vi "Us2.vi"() -> ()   [LabVIEW 2021]
panel:
  in  "\\hat b_min":dbl
  out "Us2":dbl
  out "error out":errorcluster
  in  "error in (no error)":errorcluster
  in  "z":dbl
  in  "eps":dbl
  in  "h":dbl
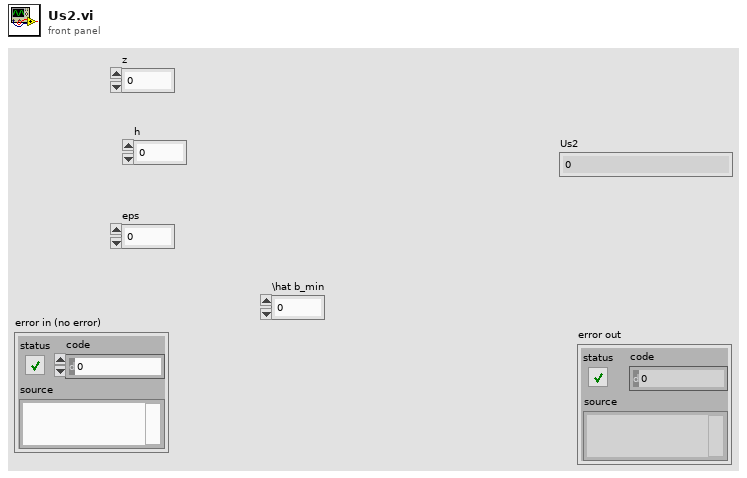
[diagram p1: front panel]
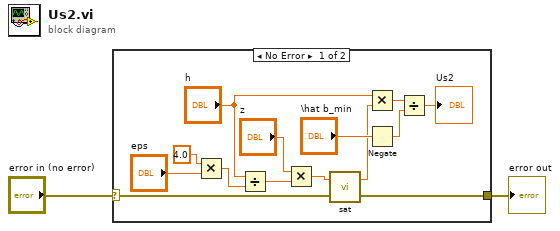
[diagram p0: block diagram]
diagram:
  n1 = case shown="No Error" "error in (no error)" {
    selector: "error in (no error)" -> [w4 w17]
    tunnel: [w3 w17] -> w1
    frame No Error {
      n2 = Multiply(x=4.0, y="eps") -> (x*y=w12:dbl)
      n3 = Divide(x="h", y=w12) -> (x/y=w11:dbl)
      n4 = Multiply(x="z", y=w11) -> (x*y=w9:dbl)
      n5 = call "sat.vi"("error in (no error)"=w4, "x"=w9) -> ("error out"=w3:errorcluster, "sat(x)"=w8:dbl)
      n6 = Multiply(x="h", y=w8) -> (x*y=w6:dbl)
      n7 = Negate(x="\\hat b_min") -> (-x=w15:dbl)
      n8 = Divide(x=w6, y=w15) -> (x/y=→"Us2":dbl)
    }
    frame Error {
    }
  }
  "error out" <- w1
